vi "Recall Save Instrument Settings.vi"(8 "error in (no error)":errorcluster, 9 "Setup Memory Location (0)":i32, 10 "Operation (0: Recall)":u16(ring) items=["Recall", "Save"], 11 "VISA resource name":refnum<visa-resource-name>) -> (0 "error out":errorcluster, 3 "VISA resource name out":refnum<visa-resource-name>)   [LabVIEW 2016, in "Tektronix AFG 1000 Series.lvlib"]
doc: "Recalls or saves the current setting of the instrument."
uses:
  Tektronix AFG 1000 Series.lvlib
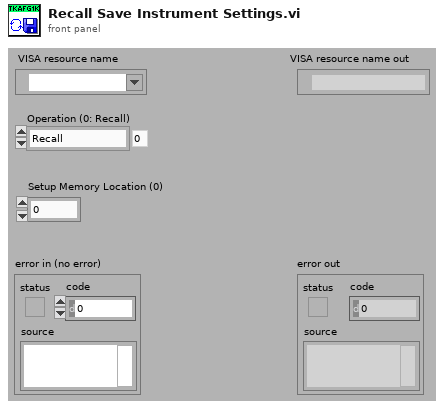
[diagram p1: front panel]
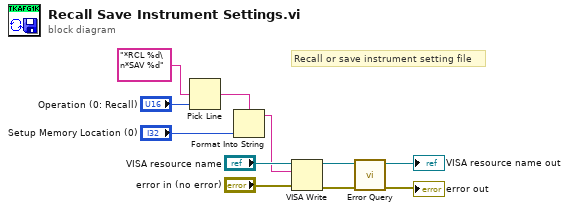
[diagram p0: block diagram]
diagram:
  # "Recall or save instrument setting file"
  n1 = Pick Line(multi-line string="*RCL %d\n*SAV %d" ("string (\"\")"), line index="Operation (0: Recall)") -> (output string=w1:string)  [unwired: 1 in]
  n2 = Format Into String(format string=w1, "Setup Memory Location (0)") -> (resulting string=w4:string)  [unwired: 2 in, 1 out]
  n3 = VISA Write(VISA resource name="VISA resource name", write buffer=w4, error in (no error)="error in (no error)") -> (VISA resource name out=w8:refnum<visa-resource-name>, error out=w7:errorcluster)  [unwired: 1 out]
  n4 = call "Error Query.vi"("error in (no error)"=w7, "VISA resource name"=w8) -> ("error out"=→"error out":errorcluster, "VISA resource name out"=→"VISA resource name out":refnum<visa-resource-name>)  [unwired: 6 in, 2 out]
